vi "Clip_Rect.vi"(2 "bounds":T1, 3 "rect":T1) -> (1 "result":T1)   [LabVIEW 2012]
uses:
  <userlib>/BIAS2/subvis/ROI_rect.ctl
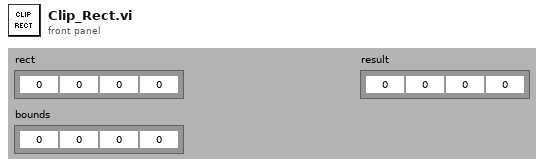
[diagram p1: front panel]
types:
  T1 = typedef "ROI_rect.ctl" = cluster{"left":i32, "top":i32, "right":i32, "bottom":i32}
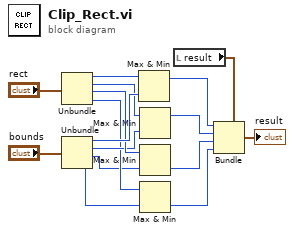
[diagram p0: block diagram]
diagram:
  n1 = Unbundle("rect") -> ("left"=w14:i32, "top"=w12:i32, "right"=w11:i32, "bottom"=w9:i32)
  n2 = Unbundle("bounds") -> ("left"=w13:i32, "top"=w10:i32, "right"=w8:i32, "bottom"=w7:i32)
  n3 = Max & Min(x=w14, y=w13) -> (max(x,y)=w5:i32)  [unwired: 1 out]
  n4 = Max & Min(x=w12, y=w10) -> (max(x,y)=w4:i32)  [unwired: 1 out]
  n5 = Max & Min(x=w11, y=w8) -> (min(x,y)=w3:i32)  [unwired: 1 out]
  n6 = Max & Min(x=w9, y=w7) -> (min(x,y)=w2:i32)  [unwired: 1 out]
  n7 = local read "result"() -> (w1:T1)
  n8 = Bundle(cluster=w1, "left"=w5, "top"=w4, "right"=w3, "bottom"=w2) -> (→"result":T1)
